vi "GA Get Capture Status.vi"(0 "nEncodeNum":i16, 1 "pClock":u32, 5 "pStatus":i16, 7 "pValue":i32, 9 "nCount":i16, 11 "error in (no error)":errorcluster caption="错误输入（无错误）") -> (3 "pClock out":u32, 4 "function return":i32, 6 "pStatus out":i16, 8 "pValue out":i32, 15 "error out":errorcluster caption="错误输出")   [LabVIEW 2015, in "GAS.lvlib"]
doc: "extern \"C\" __declspec(dllimport) int GA_GetCaptureStatus(short nEncodeNum,short *pStatus,long *pValue,short nCount=1,unsigned long *pClock=NULL);"
uses:
  <userlib>/BP_GAS/GAS.lvlib
  <userlib>/BP_GAS/GAS.dll
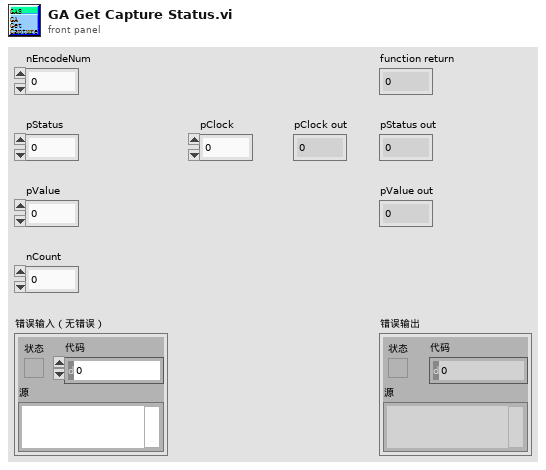
[diagram p1: front panel]
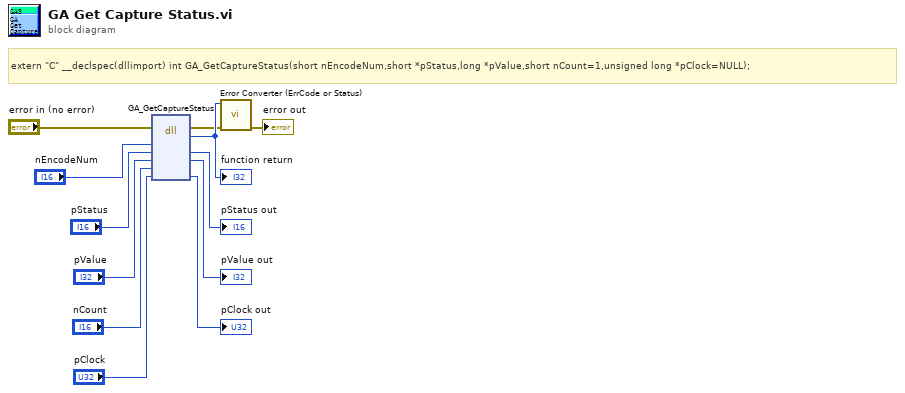
[diagram p0: block diagram]
diagram:
  # "extern \"C\" __declspec(dllimport) int GA_GetCaptureStatus(short nEncodeNum,short *pStatus,long *pValue,short nCount=1,unsigned long *pClock=NULL);"
  n1 = dll-call lib="E:/Program Files (x86)/National Instruments/LabVIEW 2015/user.lib/BP_GAS/GAS.*" fn="GA_GetCaptureStatus"(error in="error in (no error)", "nEncodeNum"="nEncodeNum", "pStatus"="pStatus", "pValue"="pValue", "nCount"="nCount", "pClock"="pClock") -> (error out=w2:errorcluster, w12:i32, "pStatus"=→"pStatus out":i16, "pValue"=→"pValue out":i32, "pClock"=→"pClock out":u32)  [unwired: 4 in, 1 out]
  "function return" <- w12
  n2 = call "Error Converter (ErrCode or Status).vi"("error in (no error)"=w2, "error code"=w12) -> ("error out"=→"error out":errorcluster)  [unwired: 9 in]
